vi "Arduino_Based_Automated_Farming_System.vi"() -> ()   [LabVIEW 2020]
panel:
  out "moisture chart":dbl(graph)
  out "water_Level chart":dbl(graph)
  out "OFF (Not Fetching Water)":bool
  out "Water Level":dbl
  out "Water Tank":dbl(slide) scale=0.0..100.0
  out "ON (Fetching Water)":bool
  out "water_level":dbl(slide) scale=0.0..100.0
  out "OFF (Not Supplying Water )":bool
  out "ON (Supplying Water to Farm)":bool
  out "Moisture Content":dbl
  out "Water Pump":u8(slide) scale=0.0..100.0
  in  "VISA resource name":refnum<visa-resource-name>
  in  "Table Control":string[][](table)
  out "moisture":dbl(knob) scale=0.0..100.0
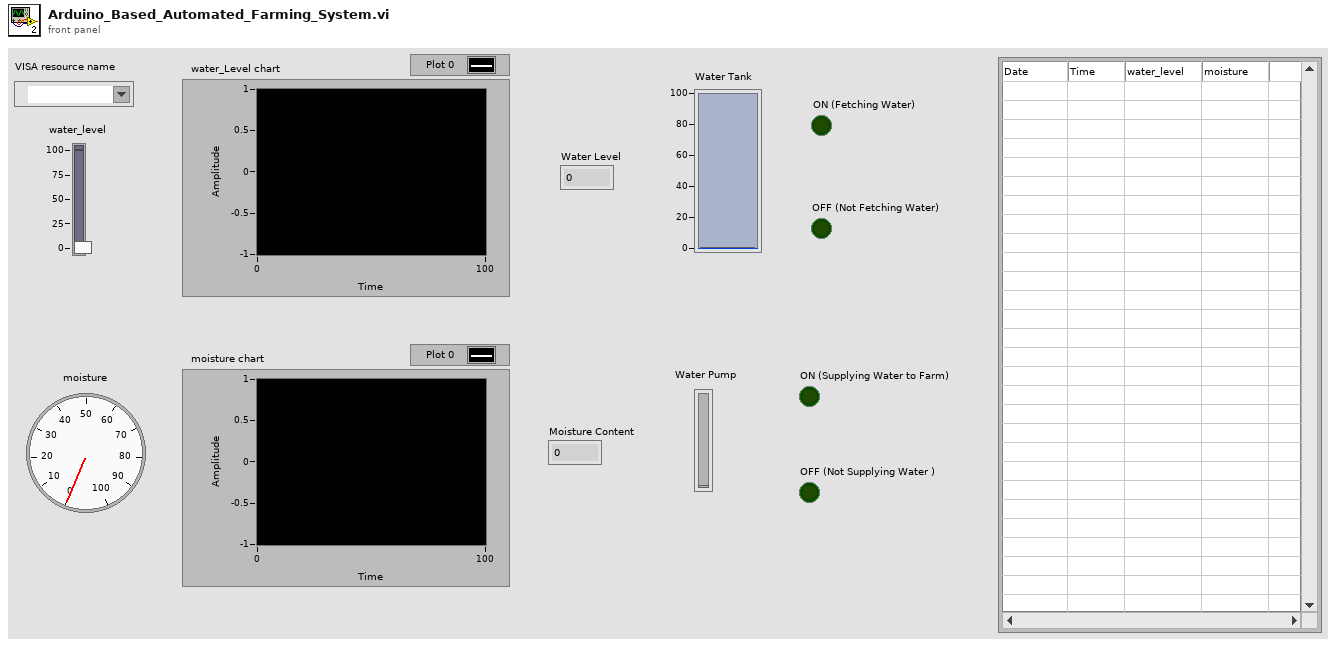
[diagram p1: front panel]
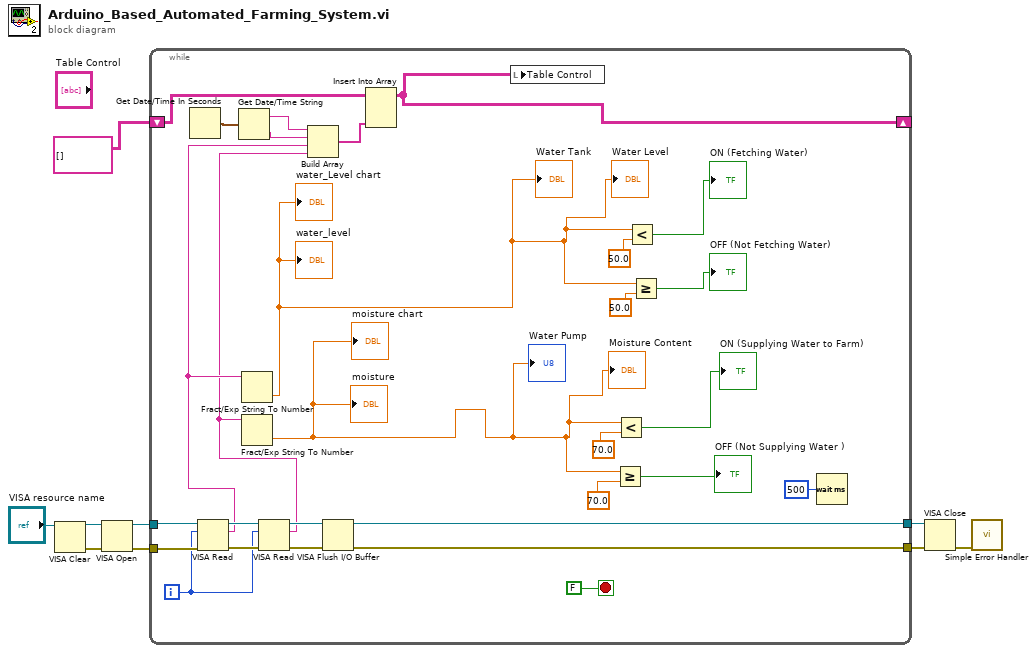
[diagram p0: block diagram]
diagram:
  n1 = VISA Clear(VISA resource name="VISA resource name") -> (VISA resource name out=w9:refnum<visa-resource-name>, error out=w8:errorcluster)  [unwired: 1 in]
  n2 = VISA Open(error in (no error)=w8, VISA resource name=w9) -> (VISA resource name=w7:refnum<visa-resource-name>, error out=w6:errorcluster)  [unwired: 3 in]
  n3 = while {
    tunnel: w7 -> [w38]
    tunnel: w6 -> [w37]
    tunnel: [w36] -> w4
    tunnel: [w31] -> w3
    shift-right: [w28] -> _
    shift-left: string[][] [] -> [w29]
    i -> [w27]
    stop <- FALSE stop-if-true
    n4 = Get Date/Time In Seconds() -> (seconds since 1Jan1904=w26:timestamp)
    n5 = VISA Read(VISA resource name=w38, byte count=w27, error in (no error)=w37) -> (VISA resource name out=w35:refnum<visa-resource-name>, read buffer=w23:string, error out=w33:errorcluster)  [unwired: 1 out]
    n6 = Get Date/Time String(seconds (now)=w26) -> (date string=w25:string, time string=w24:string)  [unwired: 2 in]
    n7 = Fract/Exp String To Number(string=w23) -> (number=w11:dbl)  [unwired: 3 in, 1 out]
    "water_level" <- w11
    "Water Tank" <- w11
    "Water Level" <- w11
    "water_Level chart" <- w11
    n8 = VISA Read(VISA resource name=w35, byte count=w27, error in (no error)=w33) -> (VISA resource name out=w34:refnum<visa-resource-name>, read buffer=w22:string, error out=w32:errorcluster)  [unwired: 1 out]
    n9 = Fract/Exp String To Number(string=w22) -> (number=w10:dbl)  [unwired: 3 in, 1 out]
    "moisture" <- w10
    "Water Pump" <- w10
    "Moisture Content" <- w10
    "moisture chart" <- w10
    n10 = Build Array(w25, w24, w23, w22) -> (w21:string[])
    n11 = VISA Flush I/O Buffer(VISA resource name=w34, error in (no error)=w32) -> (VISA resource name out=w36:refnum<visa-resource-name>, error out=w31:errorcluster)  [unwired: 1 in]
    n12 = Insert Into Array(array=w29, new element=w21) -> (w28:string[][])  [unwired: 2 in]
    n13 = local write "Table Control"(w28) -> ()
    n14 = Greater Or Equal?(x=w10, y=70.0) -> (x >= y?=→"OFF (Not Supplying Water )":bool)
    n15 = Less?(x=w10, y=70.0) -> (x < y?=→"ON (Supplying Water to Farm)":bool)
    n16 = Less?(x=w11, y=50.0) -> (x < y?=→"ON (Fetching Water)":bool)
    n17 = Greater Or Equal?(x=w11, y=50.0) -> (x >= y?=→"OFF (Not Fetching Water)":bool)
    n18 = Wait (ms)(milliseconds to wait=u32 500) -> ()  [unwired: 1 out]
  }
  n19 = VISA Close(VISA resource name=w4, error in (no error)=w3) -> (error out=w5:errorcluster)
  n20 = call <vilib>:"Simple Error Handler.vi"("error in (no error)"=w5) -> ()  [unwired: 4 in, 5 out]
